vi "ObstacleBallRadius.vi"(7 "ignoreBall?":bool, 9 "Goal":dbl[](array[numeric]), 10 "Initial State":dbl[](array[numeric]), 11 "ball":dbl[](array[numeric])) -> (2 "obstacle enemy radius":dbl)   [LabVIEW 2020]
uses:
  <vilib>/Analysis/_algsub.llb/Real Vector Norm.vi
  <vilib>/Analysis/NI_AALPro.lvlib
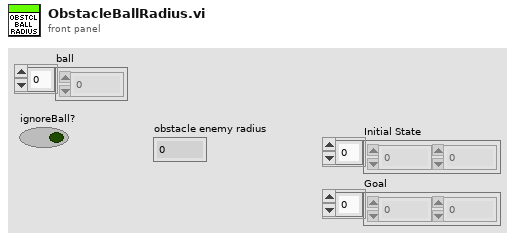
[diagram p1: front panel]
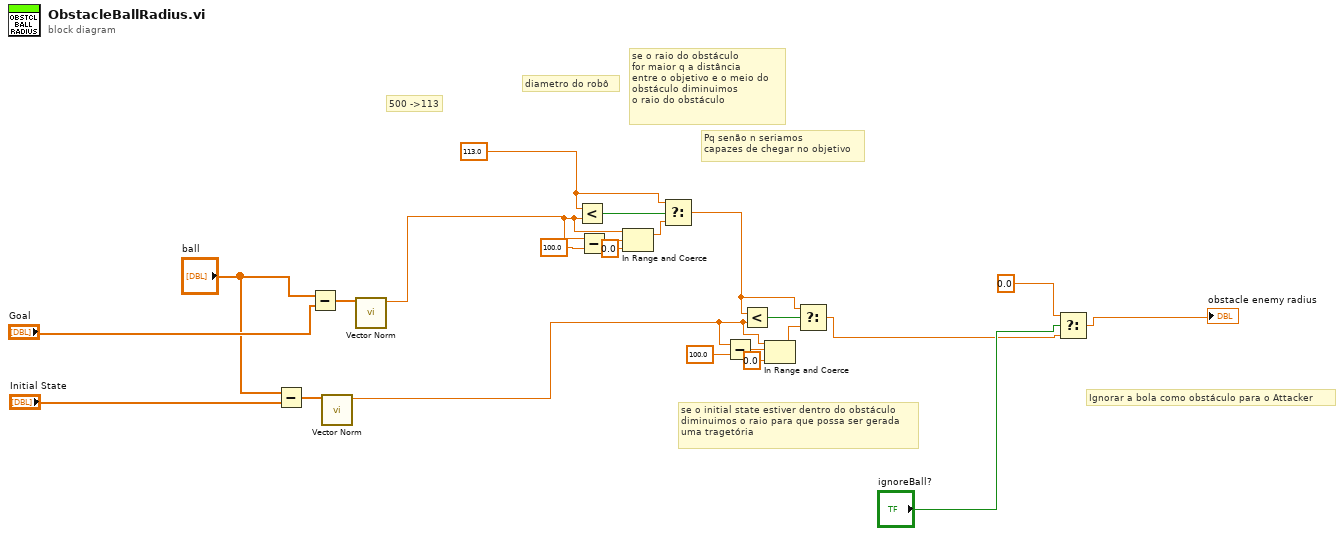
[diagram p0: block diagram]
diagram:
  w14 = 113.0 ("x")
  # "500 ->113"
  # "Ignorar a bola como obstáculo para o Attacker"
  # "se o initial state estiver dentro do obstáculo\ndiminuimos o raio para que possa ser gerada\numa tragetória"
  # "diametro do robô"
  # "Pq senão n seriamos\ncapazes de chegar no objetivo"
  # "se o raio do obstáculo\nfor maior q a distância \nentre o objetivo e o meio do \nobstáculo diminuimos \no raio do obstáculo"
  n1 = Subtract(x="ball", y="Initial State") -> (x-y=w20:dbl[])
  n2 = Subtract(x="ball", y="Goal") -> (x-y=w23:dbl[])
  n3 = call-poly <vilib>:"Vector Norm.vi"("Input Vector"=w20) -> ("norm"=w7:dbl)  [unwired: 9 in, 1 out]
  n4 = call-poly <vilib>:"Vector Norm.vi"("Input Vector"=w23) -> ("norm"=w12:dbl)  [unwired: 9 in, 1 out]
  n5 = Less?(x=w14, y=w12) -> (x < y?=w22:bool)
  n6 = Subtract(x=w12, y=100.0) -> (x-y=w13:dbl)
  n7 = In Range and Coerce(upper limit=w12, x=w13, lower limit=0.0) -> (coerced(x)=w10:dbl)  [unwired: 1 out]
  n8 = Select(t=w14, s=w22, f=w10) -> (s? t:f=w17:dbl)
  n9 = Subtract(x=w7, y=100.0) -> (x-y=w8:dbl)
  n10 = Less?(x=w17, y=w7) -> (x < y?=w18:bool)
  n11 = In Range and Coerce(upper limit=w7, x=w8, lower limit=0.0) -> (coerced(x)=w6:dbl)  [unwired: 1 out]
  n12 = Select(t=w17, s=w18, f=w6) -> (s? t:f=w2:dbl)
  n13 = Select(t=0.0, s="ignoreBall?", f=w2) -> (s? t:f=→"obstacle enemy radius":dbl)
